vi "KeithleyMeter Init.vi"(7 "Source-meter":bool, 8 "Error In":errorcluster, 9 "Prefix command":string, 10 "Parameters":T1={"Range (-1: auto)"=2.0, "Integration Time (NPLCs)"=0.1, "Function"=enum."VOLTAGE", "W Offset comp"=FALSE, "4-wire W"=FALSE, "Scale"=1.0, "Offset"=0.0} {"Integration Time (NPLCs)" min=0.01 max=10.0 step=0.01 format="%.2f"}, 11 "VISA resource name":refnum<visa-resource-name>) -> (0 "Error Out":errorcluster, 3 "VISA resource name out":refnum<visa-resource-name>)   [LabVIEW 2019]
uses:
  Keithley Meter Parameters.ctl
  KeithleyMeter Function.ctl
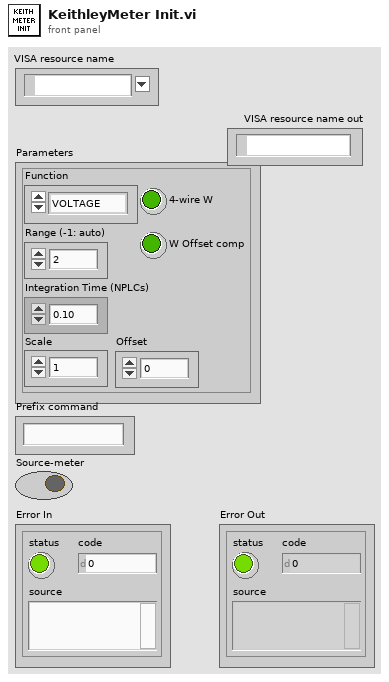
[diagram p1: front panel]
types:
  T1 = typedef "Keithley Meter Parameters.ctl" = cluster{"Range (-1: auto)":dbl, "Integration Time (NPLCs)":dbl, "Function":T2, "W Offset comp":bool, "4-wire W":bool, "Scale":dbl, "Offset":dbl}
  T2 = typedef "KeithleyMeter Function.ctl" = enum16{"VOLTAGE", "CURRENT", "RESISTANCE"}
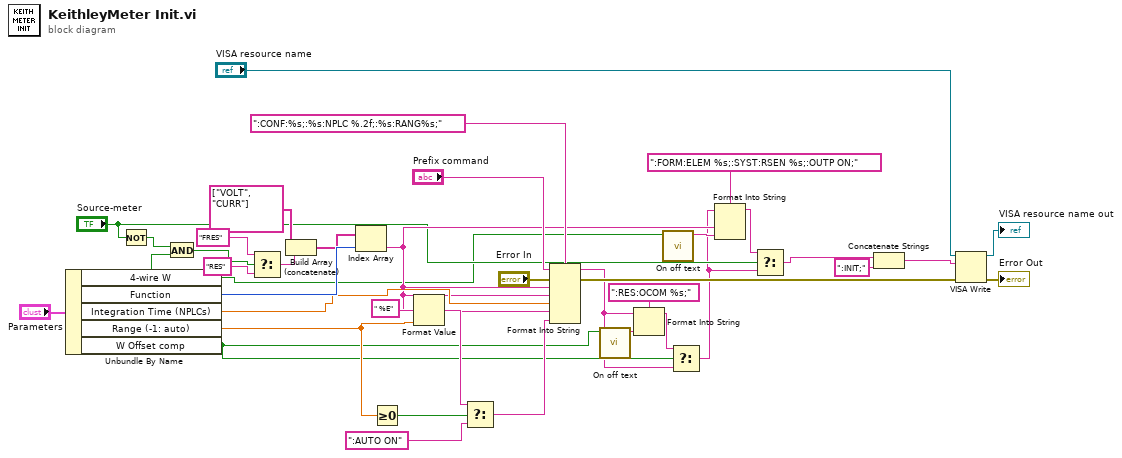
[diagram p0: block diagram]
diagram:
  n1 = Unbundle By Name("Parameters") -> ("4-wire W"=w8:bool, "Function"=w25:T2, "Integration Time (NPLCs)"=w24:dbl, "Range (-1: auto)"=w28:dbl, "W Offset comp"=w3:bool)
  n2 = Not(x="Source-meter") -> (.not. x?=w14:bool)
  n3 = And(x=w14, y=w8) -> (x .and. y?=w12:bool)
  n4 = Select(t="FRES", s=w12, f="RES") -> (s? t:f=w10:string)
  n5 = Build Array (concatenate)(string[] ["VOLT", "CURR"], w10) -> (w13:string[])
  n6 = Index Array(array=w13, index=w25) -> (element=w18:string)
  n7 = Greater Or Equal To 0?(x=w28) -> (x >= 0?=w31:bool)
  n8 = Format Value(format string=" %E", value (0)=w28) -> (output string=w29:string)  [unwired: 1 in]
  n9 = Select(t=w29, s=w31, f=":AUTO ON" ("output string")) -> (s? t:f=w23:string)
  n10 = Format Into String(format string=":CONF:%s;:%s:NPLC %.2f;:%s:RANG%s;", initial string="Prefix command", error in="Error In", w18, w18, w24, w18, w23) -> (resulting string=w1:string, error out=w35:errorcluster)
  n11 = call "On off text.vi"("ON/OFF"=w3) -> ("ON/OFF"=w2:string)  [unwired: 10 in]
  n12 = Format Into String(format string=":RES:OCOM %s;", initial string=w1, w2) -> (resulting string=w6:string)  [unwired: 1 in, 1 out]
  n13 = call "On off text.vi"("ON/OFF"=w8) -> ("ON/OFF"=w7:string)  [unwired: 10 in]
  n14 = Select(t=w6, s=w3, f=w1) -> (s? t:f=w5:string)
  n15 = Format Into String(format string=":FORM:ELEM %s;:SYST:RSEN %s;:OUTP ON;", initial string=w5, w18, w7) -> (resulting string=w17:string)  [unwired: 1 in, 1 out]
  n16 = Select(t=w17, s="Source-meter", f=w5) -> (s? t:f=w16:string)
  n17 = Concatenate Strings(w16, ":INIT;") -> (w21:string)
  n18 = VISA Write(VISA resource name="VISA resource name", write buffer=w21, error in (no error)=w35) -> (VISA resource name out=→"VISA resource name out":refnum<visa-resource-name>, error out=→"Error Out":errorcluster)  [unwired: 1 out]
